vi "get wheel popup db.vi"(2 "wheel number":dbl, 3 "Ring":u16(ring)=1 items=["10Be"=1, "14C"=2, "26Al"=3, "36Cl"=5, "41Ca"=6, "129I"=7]) -> (0 "wheel number 2":dbl, 1 "Ring 2":u16)   [LabVIEW 2016]
panel:
  in  "Boolean":bool
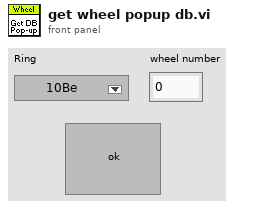
[diagram p1: front panel]
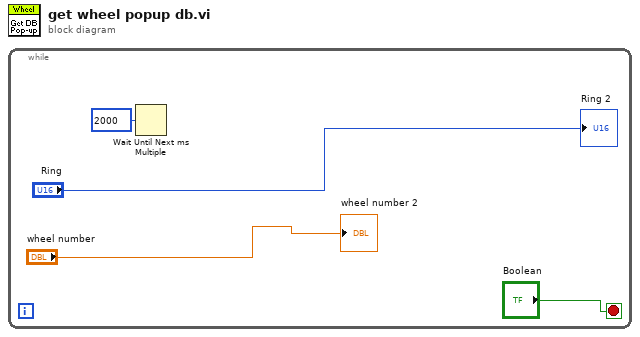
[diagram p0: block diagram]
diagram:
  n1 = while {
    stop <- "Boolean" stop-if-true
    n2 = Wait Until Next ms Multiple(millisecond multiple=u32 2000) -> ()  [unwired: 1 out]
    "wheel number 2" <- "wheel number"
    "Ring 2" <- "Ring"
  }
